vi "test I64-I16 Array.vi"() -> ()   [LabVIEW 2013]
uses:
  <vilib>/addons/_JKI Toolkits/Caraya/classes/Assert/Assert Equal Value_Variant.vi
  <vilib>/addons/_JKI Toolkits/Caraya/classes/Test/Test.lvclass
  <vilib>/addons/_JKI Toolkits/Caraya/classes/Assert/Assert.lvclass
panel:
  out "error out":errorcluster
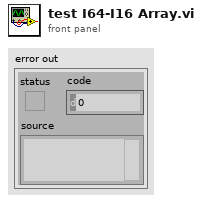
[diagram p1: front panel]
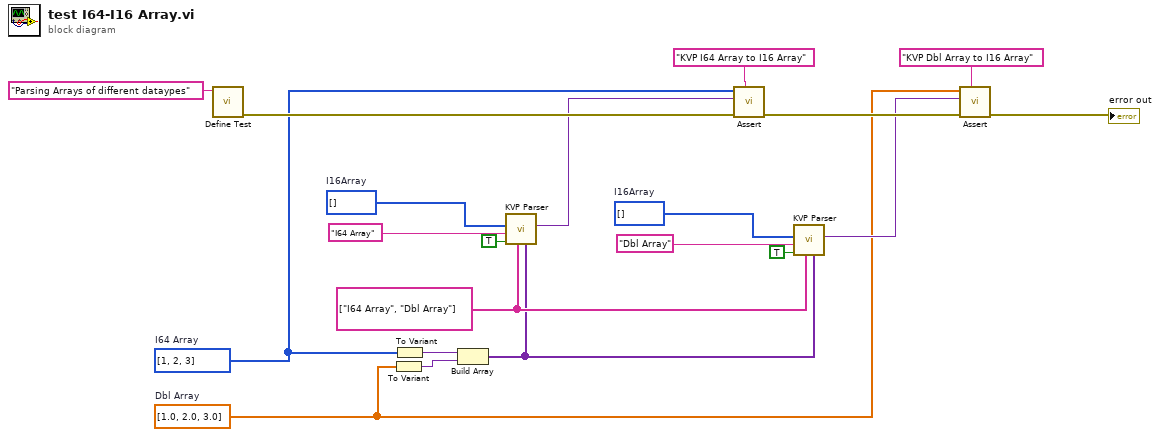
[diagram p0: block diagram]
diagram:
  w11 = i16[] []  # I16Array
  w2 = dbl[] [1.0, 2.0, 3.0]  # Dbl Array
  w8 = string[] ["I64 Array", "Dbl Array"]
  w14 = i64[] [1, 2, 3]  # I64 Array
  w12 = i16[] []  # I16Array
  n1 = call <vilib>:"Define Test.vi"("Label (VI Title)"="Parsing Arrays of different dataypes") -> ("error out"=w16:errorcluster)  [unwired: 10 in]
  n2 = To Variant(anything=w2) -> (Variant=w1:variant)
  n3 = To Variant(anything=w14) -> (Variant=w20:variant)
  n4 = Build Array(w20, w1) -> (w7:variant[])
  n5 = call "KVP Parser.vi"("Values"=w7, "Keys"=w8, "Strict type matching? (F)"=TRUE, "Default Value Name (empty: label)"="I64 Array", "Default Value"=w12) -> ("Value"=w15:variant)  [unwired: 3 in, 3 out]
  n6 = call-poly <vilib>:"Assert.vi"("Label"="KVP I64 Array to I16 Array" ("Label (VI Title)"), "error in (no error)"=w16, "Y"=w15, "X"=w14) -> ("error out"=w5:errorcluster)  [unwired: 7 in]
  n7 = call "KVP Parser.vi"("Values"=w7, "Keys"=w8, "Strict type matching? (F)"=TRUE, "Default Value Name (empty: label)"="Dbl Array", "Default Value"=w11) -> ("Value"=w3:variant)  [unwired: 3 in, 3 out]
  n8 = call-poly <vilib>:"Assert.vi"("Label"="KVP Dbl Array to I16 Array" ("Label (VI Title)"), "error in (no error)"=w5, "Y"=w3, "X"=w2) -> ("error out"=→"error out":errorcluster)  [unwired: 7 in]
